vi "Untitled 2.vi"() -> ()   [LabVIEW 2014]
panel:
  out "millisecond timer value":u32
  in  "stop":bool
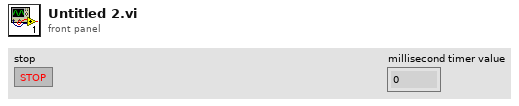
[diagram p1: front panel]
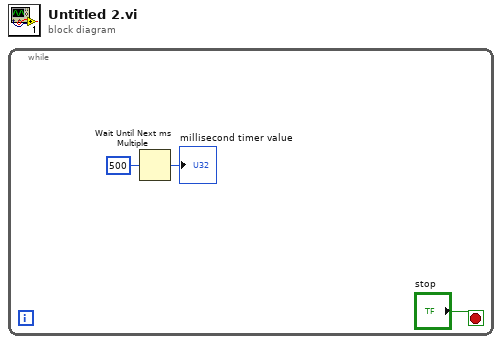
[diagram p0: block diagram]
diagram:
  n1 = while {
    stop <- "stop" stop-if-true
    n2 = Wait Until Next ms Multiple(millisecond multiple=u32 500) -> (millisecond timer value=→"millisecond timer value":u32)
  }
